vi "Read configuration.vi"(7 "force loading?":bool=TRUE, 8 "error in (no error)":errorcluster, 11 "TomoConversion in":refnum<class "TomoConversion.lvclass">) -> (0 "error out":errorcluster, 3 "TomoConversion out":refnum<class "TomoConversion.lvclass">)   [LabVIEW 2012, in "TomoConversion.lvclass"]
doc: "Reads the XML-based configuration file and populates the configuration cluster accordingly. Configuration file name is <component ID>.xml."
uses:
  TomoConversion.lvclass
  <vilib>/Distrio/Murmex/Murmex/Murmex.lvclass
  TomoConversion.lvclass/TomoConversion.ctl
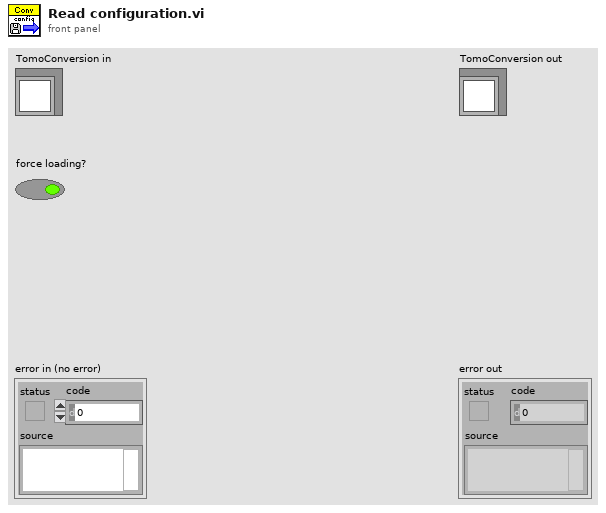
[diagram p1: front panel]
types:
  T1 = typedef "TomoConversion.lvclass/configuration_cluster.ctl" = cluster{"conversion directory path":path, "auxiliary director path":path}
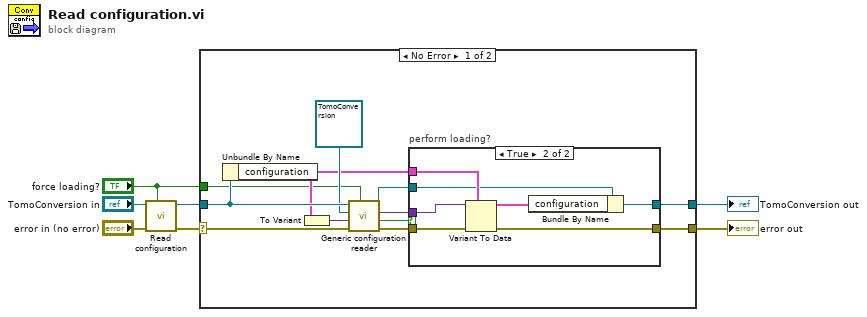
[diagram p0: block diagram]
diagram:
  n1 = call-parent "Read configuration.vi"("force loading?"="force loading?", "error in (no error)"="error in (no error)", "Murmex in"="TomoConversion in") -> ("error out"=w5:errorcluster, "Murmex out"=w4:refnum<class "TomoConversion.lvclass">)  [unwired: 7 in]
  n2 = case shown="No Error" w5 {
    selector: w5 -> [w19 w29]
    tunnel: w4 -> [w18 w30]
    tunnel: "force loading?" -> [w8 _]
    tunnel: [w10 w29] -> w2
    tunnel: [w9 w30] -> w1
    frame No Error {
      n3 = Unbundle By Name(w18) -> ("configuration"=w12:T1)
      n4 = To Variant(anything=w12) -> (Variant=w17:variant)
      n5 = call <vilib>:"Generic configuration reader.vi"("force loading?"=w8, "error in (no error)"=w19, "configuration cluster variant"=w17, "inheritance level"=refnum<class "TomoConversion.lvclass"> refnum ("TomoConversion.lvclass"), "Murmex in"=w18) -> ("error out"=w13:errorcluster, "loaded?"=w15:bool, "configuration data (variant)"=w14:variant, "Murmex out"=w11:refnum<class "TomoConversion.lvclass">)  [unwired: 3 in]
      n6 = case "perform loading?" shown="True" w15 {
        tunnel: w14 -> [_ w27]
        tunnel: w13 -> [w21 w28]
        tunnel: w12 -> [_ w26]
        tunnel: w11 -> [w20 w25]
        tunnel: [w21 w23] -> w10
        tunnel: [w20 w22] -> w9
        frame False {
        }
        frame True {
          n7 = Variant To Data(error in=w28, type=w26, Variant=w27) -> (data=w24:T1, error out=w23:errorcluster)
          n8 = Bundle By Name(cluster=w25, "configuration"=w24) -> (w22:refnum<class "TomoConversion.lvclass">)
        }
      }
    }
    frame Error {
    }
  }
  "error out" <- w2
  "TomoConversion out" <- w1
